vi "Control_ReadButton0.vi"(2 "DetectRisingEdge(F)":bool) -> (16 "ButtonPressed":bool)   [LabVIEW 2018]
uses:
  <vilib>/rvi/eio/common/nirviEmuTemplateMethod_errors.vi
  <vilib>/eio/EIONode/EIONode.xnode
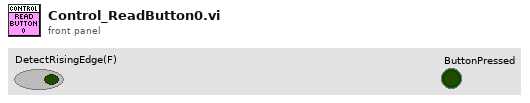
[diagram p1: front panel]
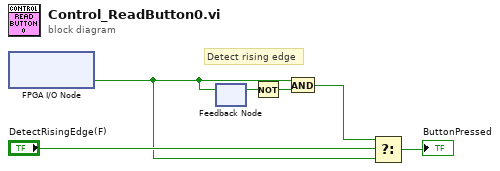
[diagram p0: block diagram]
diagram:
  # "Detect rising edge"
  n1 = xnode "FPGA I/O Node"() -> ("Button0"=w1:bool)  [unwired: 1 in, 1 out]
  n2 = feedback #1() -> (w6:bool)  [unwired: 1 in]
  n3 = feedback-in #1(w1) -> ()
  n4 = Not(x=w6) -> (.not. x?=w5:bool)
  n5 = And(x=w1, y=w5) -> (x .and. y?=w3:bool)
  n6 = Select(t=w3, s="DetectRisingEdge(F)", f=w1) -> (s? t:f=→"ButtonPressed":bool)
